vi "Card_in_out.vi"(8 "error in (no error)":errorcluster, 10 "Card":bool, 11 "UserConsole in":refnum<class "UserConsole.lvclass">) -> (0 "error out":errorcluster, 3 "UserConsole out":refnum<class "UserConsole.lvclass">)   [LabVIEW 2025, in "UserConsole.lvlib" / "UserConsole.lvclass"]
uses:
  UserConsole.lvclass
  <vilib>/ActorFramework/Actor/Actor.lvclass/Actor.ctl
  UserConsole.lvclass/UserConsole.ctl
  UserConsole Messages/Case-Controller Msg/Case-Controller Msg.lvclass/Case-Controller Msg.ctl
  <vilib>/ActorFramework/Message Enqueuer/Message Enqueuer.lvclass/Message Enqueuer.ctl
  Database_handler/Database_handler/Database_handler.lvclass
  UserConsole Messages/Balance_abs Msg/Balance_abs Msg.lvclass
  Database_handler/Database_handler/Database_handler.lvclass/Database_handler.ctl
  <vilib>/ActorFramework/Message Enqueuer/Enqueue.vi
  UserConsole Messages/Case-Controller Msg/Case-Controller Msg.lvclass
  <vilib>/ActorFramework/Stop Msg/Stop Msg.lvclass
  <vilib>/ActorFramework/Message Priority Queue/Priority Enqueue.vi
  DB_Global.vi
  <vilib>/ActorFramework/Actor/Actor.lvclass
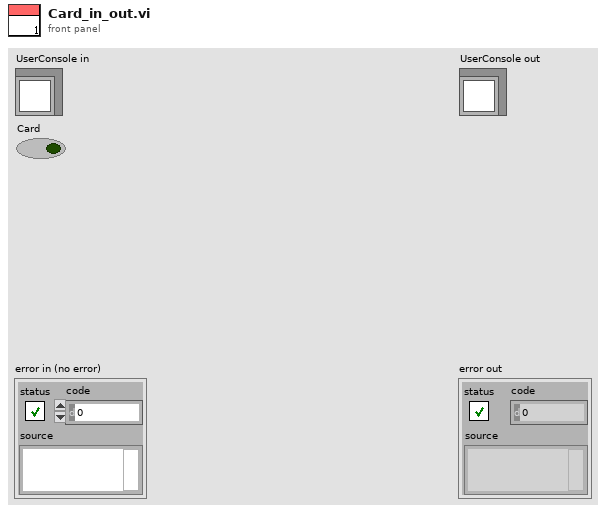
[diagram p1: front panel]
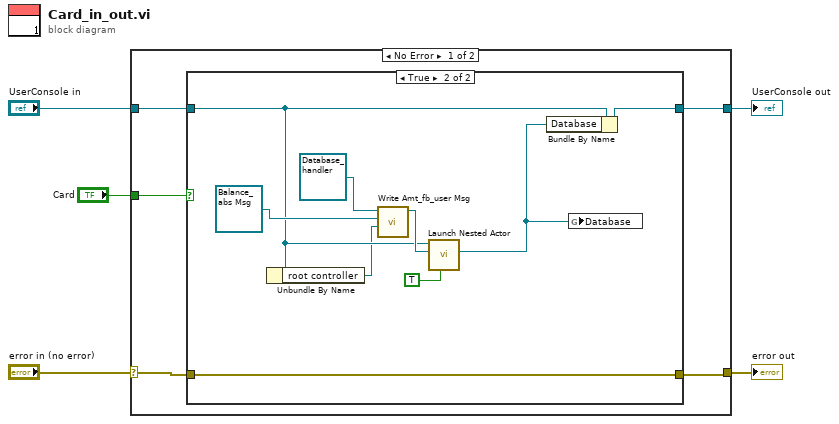
[diagram p0: block diagram]
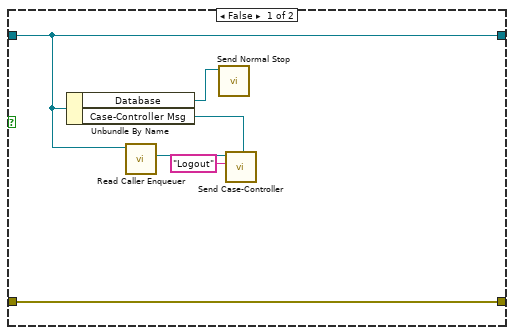
[diagram p2: hidden frame]
diagram:
  n1 = case shown="No Error" "error in (no error)" {
    selector: "error in (no error)" -> [w7 w27]
    tunnel: [w6 w27] -> w4
    tunnel: [w8 w26] -> w2
    tunnel: "UserConsole in" -> [w9 w26]
    tunnel: "Card" -> [w10 _]
    frame No Error {
      n2 = case shown="True" w10 {
        tunnel: w9 -> [w13 w18]
        tunnel: [w13 w20] -> w8
        tunnel: w7 -> [w16 w25]
        tunnel: [w16 w25] -> w6
        frame False {
          n3 = Unbundle By Name(w13) -> ("Database"=w15:refnum<class "Message Enqueuer.lvclass">, "Case-Controller Msg"=w12:refnum<class "Case-Controller Msg.lvclass">)
          n4 = call <vilib>:"Read Caller Enqueuer.vi"("Actor"=w13) -> ("Caller Enqueuer"=w14:refnum<class "Message Enqueuer.lvclass">)  [unwired: 10 in]
          n5 = call <vilib>:"Send Normal Stop.vi"("Message Enqueuer"=w15) -> ()  [unwired: 10 in, 1 out]
          n6 = call "Send Case-Controller.vi"("Message Type"=w12, "Controller Case"="Logout", "Message Enqueuer"=w14) -> ()  [unwired: 7 in, 2 out]
        }
        frame True {
          n7 = Unbundle By Name(w18) -> ("root controller"=w17:refnum<class "Message Enqueuer.lvclass">)
          n8 = call "Write Amt_fb_user Msg.vi"("Root Controller"=w17, "Database_handler.lvlib:Amt_fb_user Msg.lvclass"=refnum<class "Balance_abs Msg.lvclass"> refnum ("UserConsole.lvlib:Balance_abs Msg.lvclass"), "Database_handler in"=refnum<class "Database_handler.lvclass"> refnum ("Database_handler.lvlib:Database_handler.lvclass")) -> ("Database_handler out"=w24:refnum<class "Database_handler.lvclass">)  [unwired: 8 in]
          n9 = call <vilib>:"Launch Nested Actor.vi"("Open Actor Core front panel? (F)"=TRUE, "Nested Actor"=w24, "Caller Actor in"=w18) -> ("Nested Actor's Enqueuer"=w19:refnum<class "Message Enqueuer.lvclass">)  [unwired: 6 in, 2 out]
          n10 = Bundle By Name(cluster=w18, "Database"=w19) -> (w20:refnum<class "UserConsole.lvclass">)
          n11 = global write "DB_Global.vi" "Database"(w19) -> ()
        }
      }
    }
    frame Error {
    }
  }
  "error out" <- w4
  "UserConsole out" <- w2
